vi "Msg Create Message Queue.vi"(5 "max queue size (-1, unlimited)":i32=-1, 6 "error in (no error)":errorcluster, 7 "create if not found? (T)":bool=TRUE, 9 "name (unnamed)":string) -> (0 "error out":errorcluster, 1 "created new?":bool, 3 "queue out":refnum<queue>)   [LabVIEW 2014]
doc: "Create a message queue that enables posting of events to a standard event loop. Use Msg Get Message.vi to retrieve the messages in that loop.\n\nThis is part of the Msg suite, intended to make messaging architectures in LabVIEW\nSee the template \"Message Based Application Template.vi\" for normal usage.\n\nCopyright 2005-2016 Jason Sommerville\n\nThis VI may be freely used, modified or distributed under the BSD license."
uses:
  Message Cluster.ctl
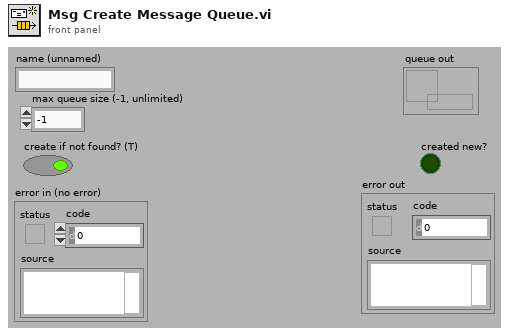
[diagram p1: front panel]
types:
  T1 = typedef "Message Cluster.ctl" = cluster{"Message":string, "Data":variant, "Response Notifier":refnum<notifier>}
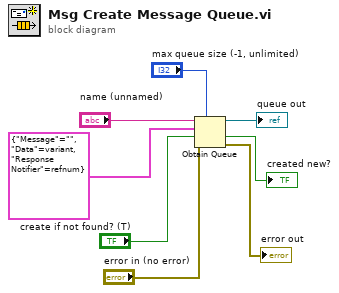
[diagram p0: block diagram]
diagram:
  n1 = Obtain Queue(max queue size (-1, unlimited)="max queue size (-1, unlimited)", name (unnamed)="name (unnamed)", element data type=T1 {"Message"="", "Data"=variant, "Response Notifier"=refnum} ("Message Cluster"), create if not found? (T)="create if not found? (T)", error in (no error)="error in (no error)") -> (queue out=→"queue out":refnum<queue>, created new?=→"created new?":bool, error out=→"error out":errorcluster)
